vi "Trainer_Stim.vi"() -> ()   [LabVIEW 2013]
uses:
  Scanner/Database/Database.lvclass
  <instrlib>/niHWS/nihws.llb/niHWS Open File Permissions ID.ctl
  <vilib>/Analysis/5stat.llb/RMS (DBL).vi
  <vilib>/DAQmx/write.llb/DAQmx Write (Digital Bool 1Line 1Point).vi
  <vilib>/DAQmx/create/channels.llb/DAQmx Create Channel (DO-Digital Output).vi
  <instrlib>/niHWS/nihws.llb/niHWS Write Analog DBL.vi
  <vilib>/DAQmx/miscellaneous.llb/DAQmx Fill In Error Info.vi
  <vilib>/Analysis/NI_AALPro.lvlib
  <vilib>/vision/NI_Vision_Development_Module.lvlib
panel:
  in  "Boolean":bool
  in  "liquid_type":string(combo)="water"
  out "error out":errorcluster
  out "error IO":errorcluster
  in  "Rec":bool
  out "Licks":bool
  out "Last timestamp (ms)":dbl format="%#_14g"
  in  "mouse_id":dbl
  out "Delivered microL":dbl
  in  "microL/pulse":dbl=8.8
  in  "ITI":u32=500
  out "# of rewards":dbl
  in  "Calibrate":bool
  in  "Reward!":bool
  out "Water":bool
  in  "Pulse time":u32=500
  out "Correct lick":bool
  in  "% decrease Thr":dbl=10.0
  out "rms value":dbl format="%0.2f"
  out "Waveform Chart":dynamicdata(graph)
  in  "stop (F)":bool
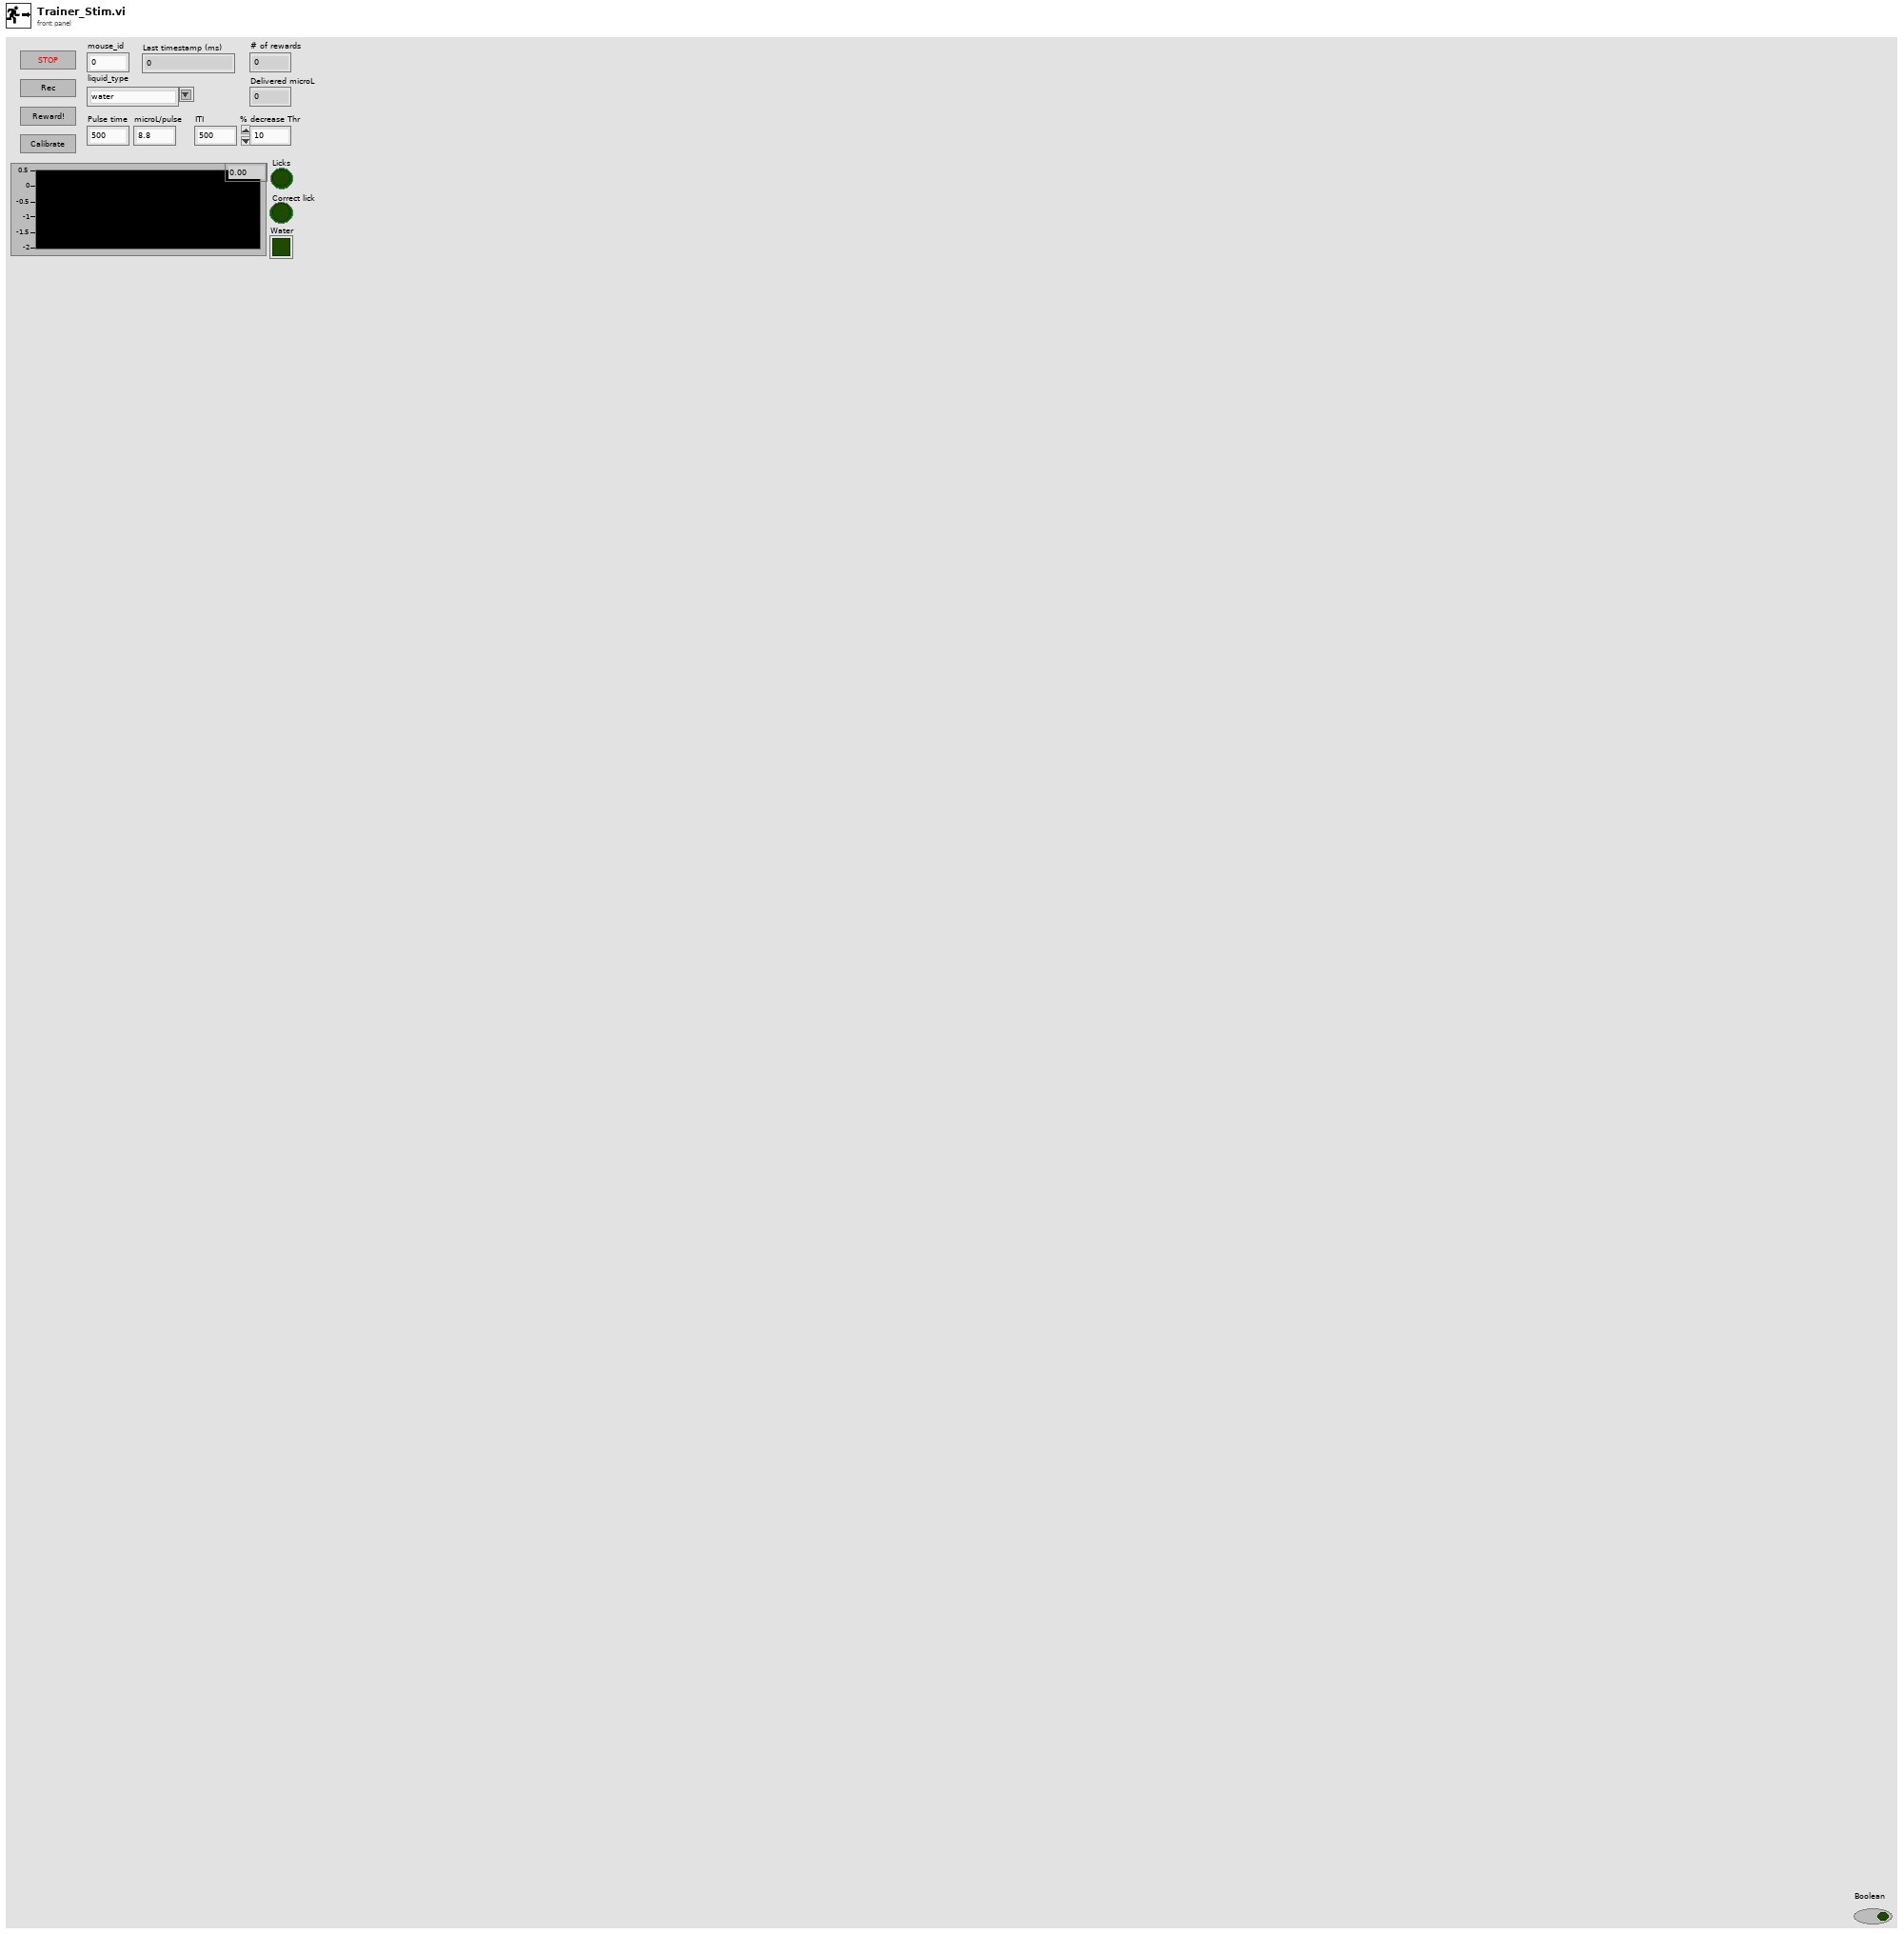
[diagram p1: front panel]
types:
  T1 = typedef "niHWS Open File Permissions ID.ctl" = enum32{"Read Only", "Read/Write Existing", "Read/Write/Create New", "Read/Write/Create New Always"}
  T2 = cluster{"mouse_id":dbl, "exp_date":string, "timestamp":dbl, "pulse_time":dbl, "microl_per_pulse":dbl, "liquid_type":string}
  T3 = typedef "IMAQ Image.ctl" = refnum<image>
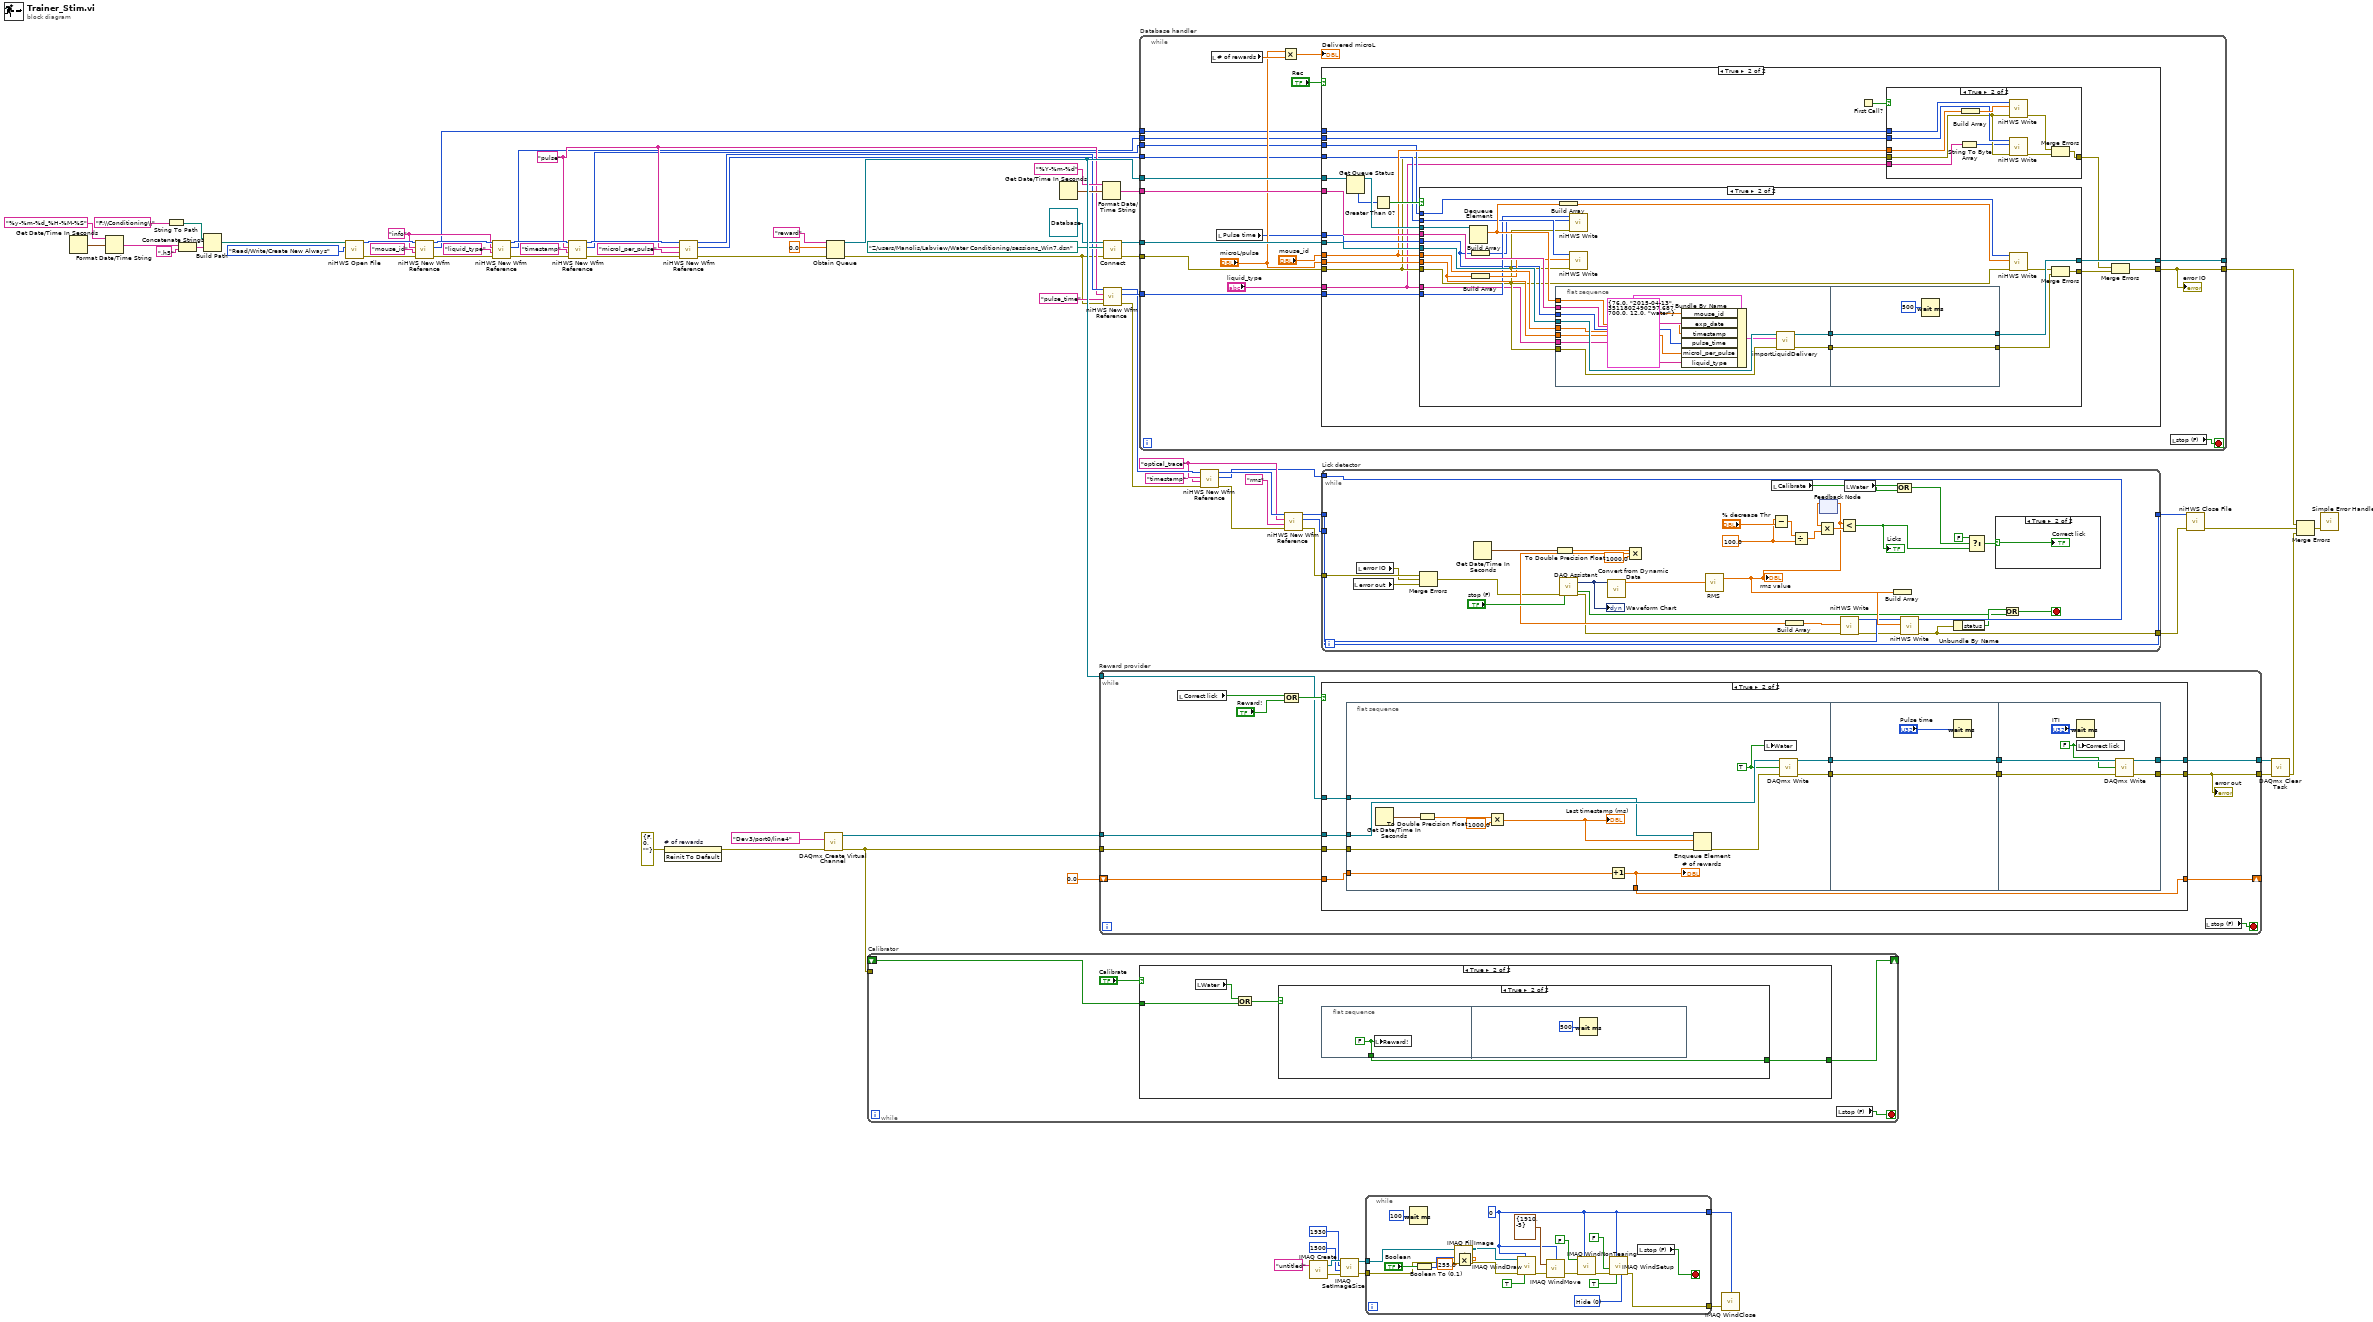
[diagram p0: block diagram]
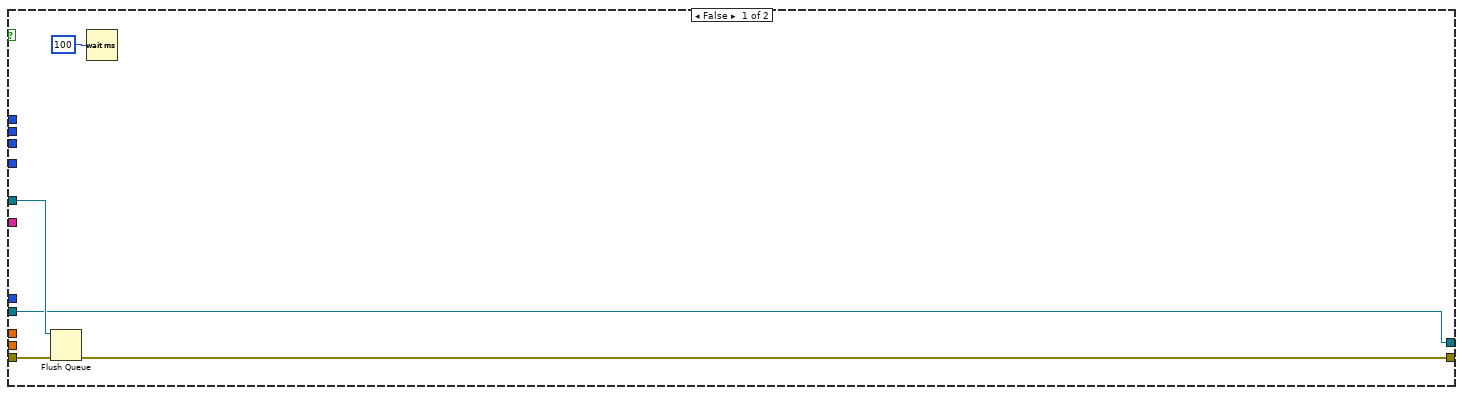
[diagram p2: hidden frame]
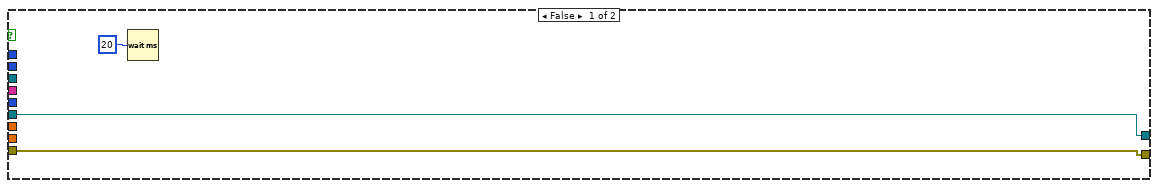
[diagram p4: hidden frame]
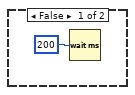
[diagram p5: hidden frame]
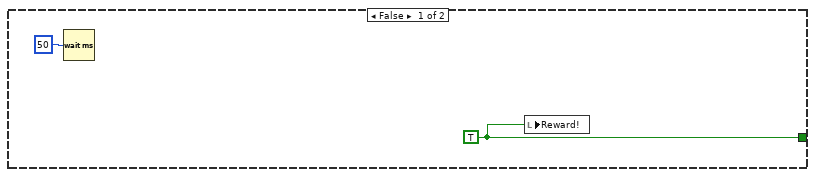
[diagram p6: hidden frame]
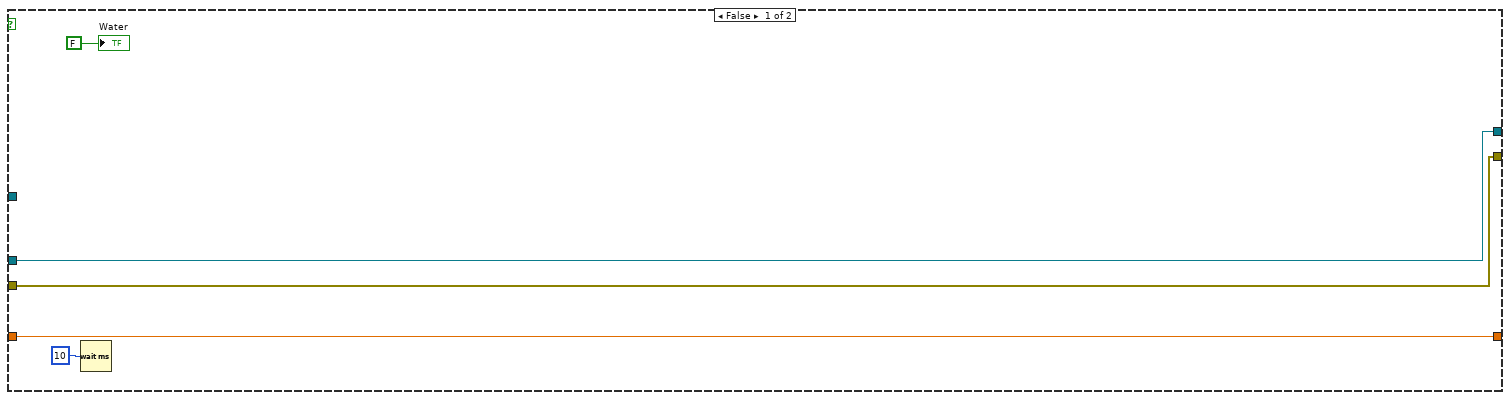
[diagram p7: hidden frame]
diagram:
  w25 = "optical_trace" ("group name (empty)")
  w36 = "pulse" ("group name (empty)")
  w45 = "info" ("group name (empty)")
  n1 = Get Date/Time In Seconds() -> (seconds since 1Jan1904=w55:timestamp)
  n2 = Format Date/Time String(time format string (%c)="%y-%m-%d_%H-%M-%S", seconds (now)=w55) -> (date/time string=w53:string)  [unwired: 1 in]
  n3 = String To Path(string="F:\\Conditioning\\" ("Default path")) -> (path=w51:path)
  n4 = Concatenate Strings(w53, ".h5" ("search string")) -> (w49:string)
  n5 = Build Path(base path=w51, name or relative path=w49) -> (appended path=w58:path)
  n6 = call <instrlib>:"niHWS Open File.vi"("permissions (0:read only)"=niHWS_Open_File_Permissions_ID."Read/Write/Create New Always", "file path"=w58) -> ("error out"=w56:errorcluster, "file handle"=w57:u32)  [unwired: 8 in]
  n7 = call <instrlib>:"niHWS New Wfm Reference.vi"("error in (no error)"=w56, "waveform name (empty)"="mouse_id", "group name (empty)"=w45, "file handle in"=w57) -> ("error out"=w47:errorcluster, "waveform reference"=w34:u32, "file handle out"=w46:u32)  [unwired: 5 in]
  n8 = call <instrlib>:"niHWS New Wfm Reference.vi"("error in (no error)"=w47, "waveform name (empty)"="liquid_type", "group name (empty)"=w45, "file handle in"=w46) -> ("error out"=w43:errorcluster, "waveform reference"=w33:u32, "file handle out"=w42:u32)  [unwired: 5 in]
  n9 = call <instrlib>:"niHWS New Wfm Reference.vi"("error in (no error)"=w43, "waveform name (empty)"="timestamp", "group name (empty)"=w36, "file handle in"=w42) -> ("error out"=w39:errorcluster, "waveform reference"=w32:u32, "file handle out"=w40:u32)  [unwired: 5 in]
  n10 = invoke on="# of rewards" class="DigNum (strict)" method="Reinit To Default"(error in=errorcluster {"status"=FALSE, "code"=0, "source"=""} ("error in (no error)")) -> (error out=w61:errorcluster)  [unwired: 2 in, 2 out]
  n11 = call <instrlib>:"niHWS New Wfm Reference.vi"("error in (no error)"=w39, "waveform name (empty)"="microl_per_pulse", "group name (empty)"=w36, "file handle in"=w40) -> ("error out"=w11:errorcluster, "waveform reference"=w31:u32, "file handle out"=w37:u32)  [unwired: 5 in]
  n12 = call-poly <vilib>:"DAQmx Create Virtual Channel.vi"("lines"=tag "Dev3/port0/line4", "error in"=w61) -> ("task out"=w75:refnum<k21>, "error out"=w18:errorcluster)  [unwired: 12 in]
  n13 = Obtain Queue(name (unnamed)="reward", element data type=0.0, error in (no error)=w11) -> (queue out=w72:refnum<queue>, error out=w10:errorcluster)  [unwired: 2 in, 1 out]
  n14 = while "Calibrator" {
    shift-right: [w79] -> _
    shift-left: _ -> [w78]
    tunnel: w18 -> [_]
    stop <- w80 stop-if-true
    n15 = case shown="True" "Calibrate" {
      tunnel: [_ w85] -> w79
      tunnel: w78 -> [_ w84]
      frame False {
        n16 = Wait (ms)(milliseconds to wait=u32 200) -> ()  [unwired: 1 out]
      }
      frame True {
        n17 = local read "Water"() -> (w82:bool)
        n18 = Or(x=w82, y=w84) -> (x .or. y?=w83:bool)
        n19 = case shown="True" w83 {
          tunnel: [w87 w88] -> w85
          frame False {
            w87 = TRUE ("Juice!")
            n20 = Wait (ms)(milliseconds to wait=u32 50) -> ()  [unwired: 1 out]
            n21 = local write "Reward!"(w87) -> ()
          }
          frame True {
            n22 = flat-sequence {
              tunnel: [w89] -> w88
              frame #0 {
                w89 = FALSE
                n23 = local write "Reward!"(w89) -> ()
              }
              frame #1 {
                n24 = Wait (ms)(milliseconds to wait=u32 500 ("value")) -> ()  [unwired: 1 out]
              }
            }
          }
        }
      }
    }
    n25 = local read "stop (F)"() -> (w80:bool)
  }
  n26 = Get Date/Time In Seconds() -> (seconds since 1Jan1904=w68:timestamp)
  n27 = while "Reward provider" {
    tunnel: w75 -> [w100]
    tunnel: [w99] -> w74
    tunnel: w18 -> [w95]
    tunnel: [w91] -> w73
    tunnel: w72 -> [w94]
    shift-right: [w93] -> _
    shift-left: 0.0 -> [w92]
    stop <- w101 stop-if-true
    n28 = local read "Correct lick"() -> (w98:bool)
    n29 = Compound Arithmetic op=OR(w98, "Reward!") -> (w97:bool)
    n30 = case shown="True" w97 {
      tunnel: w100 -> [w104 w117]
      tunnel: [w104 w116] -> w99
      tunnel: w95 -> [w103 w113]
      tunnel: [w103 w110] -> w91
      tunnel: w94 -> [_ w109]
      tunnel: w92 -> [w102 w108]
      tunnel: [w102 w107] -> w93
      frame False {
        n31 = Wait (ms)(milliseconds to wait=u32 10) -> ()  [unwired: 1 out]
        "Water" <- FALSE ("data")
      }
      frame True {
        n32 = flat-sequence {
          tunnel: w117 -> [w130]
          tunnel: [w129] -> w115
          tunnel: w113 -> [w119]
          tunnel: [w127] -> w111
          tunnel: w109 -> [w126]
          tunnel: w108 -> [w121]
          tunnel: [w120] -> w107
          tunnel: w115 -> [w132]
          tunnel: [w132] -> w114
          tunnel: [w131] -> w112
          tunnel: w111 -> [w131]
          tunnel: [w138] -> w116
          tunnel: w114 -> [w139]
          tunnel: w112 -> [w136]
          tunnel: [w135] -> w110
          frame #0 {
            w128 = TRUE ("data")
            n33 = Get Date/Time In Seconds() -> (seconds since 1Jan1904=w125:timestamp)
            n34 = To Double Precision Float(number=w125) -> (double precision float=w124:dbl)
            n35 = Multiply(x=w124, y=1000.0) -> (x*y=w122:dbl)
            "Last timestamp (ms)" <- w122
            n36 = Increment(x=w121) -> (x+1=w120:dbl)
            "# of rewards" <- w120
            n37 = Enqueue Element(queue=w126, element=w122, error in (no error)=w119) -> (error out=w118:errorcluster)  [unwired: 1 in, 2 out]
            n38 = local write "Water"(w128) -> ()
            n39 = call-poly <vilib>:"DAQmx Write.vi"("task/channels in"=w130, "data"=w128, "error in"=w118) -> ("task out"=w129:refnum<k21>, "error out"=w127:errorcluster)  [unwired: 10 in, 1 out]
          }
          frame #1 {
            n40 = Wait (ms)(milliseconds to wait="Pulse time") -> ()  [unwired: 1 out]
          }
          frame #2 {
            w134 = FALSE ("data")
            n41 = Wait (ms)(milliseconds to wait="ITI") -> ()  [unwired: 1 out]
            n42 = local write "Correct lick"(w134) -> ()
            n43 = call-poly <vilib>:"DAQmx Write.vi"("task/channels in"=w139, "data"=w134, "error in"=w136) -> ("task out"=w138:refnum<k21>, "error out"=w135:errorcluster)  [unwired: 10 in, 1 out]
          }
        }
      }
    }
    "error out" <- w91
    n44 = local read "stop (F)"() -> (w101:bool)
  }
  n45 = Format Date/Time String(time format string (%c)="%Y-%m-%d", seconds (now)=w68) -> (date/time string=w65:string)  [unwired: 1 in]
  n46 = call <instrlib>:"niHWS New Wfm Reference.vi"("error in (no error)"=w10, "waveform name (empty)"="pulse_time", "group name (empty)"=w36, "file handle in"=w37) -> ("error out"=w28:errorcluster, "waveform reference"=w30:u32, "file handle out"=w29:u32)  [unwired: 5 in]
  n47 = call-dynamic "Connect.vi"("error in (no error)"=w10, "Session"=path "Z:/users/Manolis/Labview/Water Conditioning/sessions_Win7.dsn", "Database in"=refnum<class "Database.lvclass"> refnum) -> ("error out"=w66:errorcluster, "Database out"=w67:refnum<class "Database.lvclass">)  [unwired: 7 in]
  n48 = while "Database handler" {
    tunnel: w67 -> [w157]
    tunnel: w66 -> [w155]
    tunnel: [w156] -> _
    tunnel: [w141] -> w15
    tunnel: w65 -> [w154]
    tunnel: w72 -> [w153]
    tunnel: w34 -> [w146]
    tunnel: w33 -> [w145]
    tunnel: w32 -> [w144]
    tunnel: w31 -> [w143]
    tunnel: w30 -> [w142]
    stop <- w158 stop-if-true
    n49 = local read "# of rewards"() -> (w151:dbl)
    n50 = local read "Pulse time"() -> (w148:u32)
    n51 = Multiply(x="microL/pulse", y=w151) -> (x*y=→"Delivered microL":dbl)
    n52 = case shown="True" "Rec" {
      tunnel: w157 -> [w161 w184]
      tunnel: [w161 w183] -> w156
      tunnel: [w159 w166] -> w141
      tunnel: w155 -> [w160 w168]
      tunnel: w154 -> [_ w182]
      tunnel: w153 -> [w163 w178]
      tunnel: "microL/pulse" -> [_ w177]
      tunnel: "mouse_id" -> [_ w173]
      tunnel: w148 -> [_ w176]
      tunnel: w146 -> [_ w174]
      tunnel: w145 -> [_ w172]
      tunnel: w144 -> [_ w171]
      tunnel: w143 -> [_ w170]
      tunnel: w142 -> [_ w169]
      tunnel: "liquid_type" -> [_ w164]
      frame False {
        n53 = Flush Queue(queue=w163, error in (no error)=w160) -> (error out=w159:errorcluster)  [unwired: 2 out]
        n54 = Wait (ms)(milliseconds to wait=u32 100) -> ()  [unwired: 1 out]
      }
      frame True {
        n55 = Get Queue Status(queue=w178) -> (queue out=w181:refnum<queue>, # elements in queue=w180:i32)  [unwired: 2 in, 6 out]
        n56 = Greater Than 0?(x=w180) -> (x > 0?=w179:bool)
        n57 = case shown="True" w179 {
          tunnel: w184 -> [w198 w219]
          tunnel: [w198 w218] -> w183
          tunnel: [w196 w201] -> w165
          tunnel: w168 -> [w196 w200]
          tunnel: w182 -> [_ w217]
          tunnel: w177 -> [_ w207]
          tunnel: w181 -> [_ w213]
          tunnel: w173 -> [_ w214]
          tunnel: w176 -> [_ w204]
          tunnel: w171 -> [_ w210]
          tunnel: w170 -> [_ w209]
          tunnel: w169 -> [_ w206]
          tunnel: w164 -> [_ w199]
          frame False {
            n58 = Wait (ms)(milliseconds to wait=u32 20) -> ()  [unwired: 1 out]
          }
          frame True {
            n59 = Dequeue Element(queue=w213) -> (element=w212:dbl)  [unwired: 2 in, 3 out]
            n60 = Build Array(w204) -> (w205:u32[])
            n61 = Build Array(w207) -> (w208:dbl[])
            n62 = flat-sequence {
              tunnel: w219 -> [w231]
              tunnel: w200 -> [w228]
              tunnel: w217 -> [w227]
              tunnel: w207 -> [w226]
              tunnel: [w230] -> w216
              tunnel: [w229] -> w215
              tunnel: w214 -> [w225]
              tunnel: w204 -> [w224]
              tunnel: w212 -> [w223]
              tunnel: w199 -> [w220]
              tunnel: [w233] -> w202
              tunnel: [w234] -> w218
              tunnel: w216 -> [w234]
              tunnel: w215 -> [w233]
              frame #0 {
                n63 = Bundle By Name(cluster=T2 {"mouse_id"=76.0, "exp_date"="2015-04-13", "timestamp"=3511802490297.687, "pulse_time"=700.0, "microl_per_pulse"=12.0, "liquid_type"="water"} ("Tuple"), "mouse_id"=w225, "exp_date"=w227, "timestamp"=w223, "pulse_time"=w224, "microl_per_pulse"=w226, "liquid_type"=w220) -> (w221:T2)
                n64 = call-dynamic "importLiquidDelivery.vi"("error in (no error)"=w228, "Tuple"=w221, "Database in"=w231) -> ("error out"=w229:errorcluster, "Database out"=w230:refnum<class "Database.lvclass">)  [unwired: 7 in]
              }
              frame #1 {
                n65 = Wait (ms)(milliseconds to wait=u32 500) -> ()  [unwired: 1 out]
              }
            }
            n66 = Build Array(w212) -> (w211:dbl[])
            n67 = call-poly <instrlib>:"niHWS Write.vi"("error in (no error)"=w200, "data"=w205, "waveform reference in"=w206) -> ()  [unwired: 7 in, 2 out]
            n68 = call-poly <instrlib>:"niHWS Write.vi"("error in (no error)"=w200, "data"=w208, "waveform reference in"=w209) -> ()  [unwired: 7 in, 2 out]
            n69 = call-poly <instrlib>:"niHWS Write.vi"("error in (no error)"=w200, "data"=w211, "waveform reference in"=w210) -> ("error out"=w203:errorcluster)  [unwired: 7 in, 1 out]
            n70 = Merge Errors(w203, w202) -> (w201:errorcluster)
          }
        }
        n71 = First Call?() -> (First Call?: T/F=w175:bool)
        n72 = case shown="True" w175 {
          tunnel: w174 -> [_ w195]
          tunnel: w173 -> [_ w193]
          tunnel: w172 -> [_ w192]
          tunnel: w168 -> [w185 w191]
          tunnel: [w185 w188] -> w167
          tunnel: w164 -> [_ w187]
          frame False {
          }
          frame True {
            n73 = String To Byte Array(string=w187) -> (unsigned byte array=w186:u8[])
            n74 = Build Array(w193) -> (w194:dbl[])
            n75 = call-poly <instrlib>:"niHWS Write.vi"("error in (no error)"=w191, "data"=w194, "waveform reference in"=w195) -> ("error out"=w190:errorcluster)  [unwired: 7 in, 1 out]
            n76 = call-poly <instrlib>:"niHWS Write.vi"("error in (no error)"=w191, "data"=w186, "waveform reference in"=w192) -> ("error out"=w189:errorcluster)  [unwired: 7 in, 1 out]
            n77 = Merge Errors(w190, w189) -> (w188:errorcluster)
          }
        }
        n78 = Merge Errors(w167, w165) -> (w166:errorcluster)
      }
    }
    "error IO" <- w141
    n79 = local read "stop (F)"() -> (w158:bool)
  }
  n80 = call <instrlib>:"niHWS New Wfm Reference.vi"("error in (no error)"=w28, "waveform name (empty)"="timestamp", "group name (empty)"=w25, "file handle in"=w29) -> ("error out"=w26:errorcluster, "waveform reference"=w21:u32, "file handle out"=w27:u32)  [unwired: 5 in]
  n81 = call <instrlib>:"niHWS New Wfm Reference.vi"("error in (no error)"=w26, "waveform name (empty)"="rms", "group name (empty)"=w25, "file handle in"=w27) -> ("error out"=w17:errorcluster, "waveform reference"=w22:u32, "file handle out"=w20:u32)  [unwired: 5 in]
  n82 = call "IMAQ Create"("Image Name"="untitled") -> ("New Image"=w8:T3, "error out"=w3:errorcluster)  [unwired: 4 in]
  n83 = while "Lick detector" {
    tunnel: w22 -> [w253]
    tunnel: w21 -> [w252]
    tunnel: w20 -> [w246]
    tunnel: [w246] -> w19
    tunnel: w17 -> [w238]
    tunnel: [w243] -> w16
    stop <- w240 stop-if-true
    w262 = 100.0 ("y")
    n84 = local read "error out"() -> (w236:errorcluster)
    n85 = local read "error IO"() -> (w239:errorcluster)
    n86 = Merge Errors(w239, w238, w236) -> (w237:errorcluster)
    n87 = Get Date/Time In Seconds() -> (seconds since 1Jan1904=w248:timestamp)
    n88 = To Double Precision Float(number=w248) -> (double precision float=w249:dbl)
    n89 = call "DAQ Assistant"("error in"=w237, "stop (F)"="stop (F)") -> ("data"=w268:dynamicdata, "stopped"=w241:bool, "error out"=w245:errorcluster)  [unwired: 14 in, 1 out]
    "Waveform Chart" <- w268
    n90 = call "Convert from Dynamic Data"("Dynamic Data Type"=w268) -> ("Array"=w267:dbl[])  [unwired: 3 in]
    n91 = Multiply(x=w249, y=1000.0) -> (x*y=w247:dbl)
    n92 = call-poly <vilib>:"RMS.vi"("X"=w267) -> ("rms value"=w251:dbl)  [unwired: 1 out]
    "rms value" <- w251
    n93 = local read "Calibrate"() -> (w260:bool)
    n94 = Subtract(x=w262, y="% decrease Thr") -> (x-y=w261:dbl)
    n95 = Build Array(w247) -> (w255:dbl[])
    n96 = Divide(x=w261, y=w262) -> (x/y=w264:dbl)
    n97 = feedback #1() -> (w266:dbl)  [unwired: 1 in]
    n98 = Multiply(x=w266, y=w264) -> (x*y=w265:dbl)
    n99 = feedback-in #1(w251) -> ()
    n100 = Less?(x=w251, y=w265) -> (x < y?=w235:bool)
    "Licks" <- w235
    n101 = call-poly <instrlib>:"niHWS Write.vi"("error in (no error)"=w245, "data"=w255, "waveform reference in"=w252) -> ("error out"=w244:errorcluster)  [unwired: 7 in, 1 out]
    n102 = local read "Water"() -> (w259:bool)
    n103 = Build Array(w251) -> (w254:dbl[])
    n104 = Compound Arithmetic op=OR(w260, w259) -> (w258:bool)
    n105 = call-poly <instrlib>:"niHWS Write.vi"("error in (no error)"=w244, "data"=w254, "waveform reference in"=w253) -> ("error out"=w243:errorcluster)  [unwired: 7 in, 1 out]
    n106 = Unbundle By Name(w243) -> ("status"=w242:bool)
    n107 = Select(t=FALSE, s=w258, f=w235) -> (s? t:f=w256:bool)
    n108 = case shown="True" w256 {
      selector: w256 -> [_ w270]
      frame False {
      }
      frame True {
        "Correct lick" <- w270
      }
    }
    n109 = Or(x=w242, y=w241) -> (x .or. y?=w240:bool)
  }
  n110 = call "IMAQ SetImageSize"("error in (no error)"=w3, "Y Resolution"=1500 ("X Resolution"), "X Resolution"=1930, "Image"=w8) -> ("error out"=w4:errorcluster, "Image Out"=w5:T3)  [unwired: 1 in]
  n111 = while {
    tunnel: w5 -> [w286]
    tunnel: w4 -> [w279]
    tunnel: [w272] -> w2
    tunnel: [w274] -> w1
    stop <- w271 stop-if-true
    w275 = 0 items=["Hide", "Show", "No change"] ("Scrollbars (No change)")
    w274 = 0 ("Window Number (0...15)")
    n112 = Wait (ms)(milliseconds to wait=u32 100) -> ()  [unwired: 1 out]
    n113 = Boolean To (0,1)(Boolean="Boolean") -> (0, 1=w281:i16)
    n114 = Multiply(x=w281, y=255.0) -> (x*y=w280:dbl)
    n115 = call "IMAQ FillImage"("error in (no error)"=w279, "Pixel Value (U8, U16, I16, Float)"=w280, "Image"=w286) -> ("error out"=w278:errorcluster, "Image Out"=w285:T3)  [unwired: 7 in]
    n116 = call "IMAQ WindDraw"("Resize to Image Size? (Y)"=TRUE, "Window Number (0...15)"=w274, "error in (no error)"=w278, "Image"=w285) -> ("error out"=w290:errorcluster)  [unwired: 6 in, 1 out]
    n117 = call "IMAQ WindMove"("Window Number (0...15)"=w274, "Coordinates (screen)"=cluster{"X Position":i32, "Y Position":i32} {"X Position"=1910, "Y Position"=-5}, "error in (no error)"=w290) -> ("error out"=w288:errorcluster)  [unwired: 2 in, 1 out]
    n118 = call "IMAQ WindNonTearing"("Window Number"=w274, "error in (no error)"=w288, "NonTearing? (True)"=FALSE) -> ("error out"=w273:errorcluster)  [unwired: 7 in, 1 out]
    n119 = call "IMAQ WindSetup"("Scrollbars (No change)"=w275, "Window is floating? (No)"=TRUE, "Window Number (0...15)"=w274, "error in (no error)"=w273, "Window has title bar? (Yes)"=FALSE) -> ("error out"=w272:errorcluster)  [unwired: 6 in]
    n120 = local read "stop (F)"() -> (w271:bool)
  }
  n121 = call "IMAQ WindClose"("Window Number (0...15)"=w1, "error in (no error)"=w2) -> ()  [unwired: 4 in, 1 out]
  n122 = call <instrlib>:"niHWS Close File.vi"("error in (no error)"=w16, "file handle"=w19) -> ("error out"=w14:errorcluster)  [unwired: 9 in]
  n123 = call <vilib>:"DAQmx Clear Task.vi"("task in"=w74, "error in"=w73) -> ("error out"=w13:errorcluster)  [unwired: 13 in]
  n124 = Merge Errors(w15, w14, w13) -> (w12:errorcluster)
  n125 = call <vilib>:"Simple Error Handler.vi"("error in (no error)"=w12) -> ()  [unwired: 4 in, 5 out]
